vi "thermo_format_custom_values.vi"(0 "temp":dbl, 1 "format prefix":string, 2 "RH":dbl, 3 "press":dbl, 4 "channel":T1={"stat"=enum."Disabled", "type"=enum."COMET Tx5xx (ethernet)", "comment"="", "tag"="", "refresh"=5.0, "IP"="", "port"=502, "VISA"="", "last readout"=timestamp(0 s since 1904-01-01), "TCP ref"=refnum, "VISA sess"="", "idn"="", "press"=0.0, "RH"=0.0, "temp"=0.0, "pres cor"=[], "RH cor"=[], "temp cor"=[], "try left"=0, "failed"=FALSE, "RTD set"=[], "RTD inv"=[], "range"=0.0, "net mode"=enum."MODBUS"} {"RTD inv" format="%.1f"; "RTD set" format="%.1f"; "temp cor" format="%.1f"; "RH cor" format="%.1f"; "pres cor" format="%.1f"; "refresh" min=0.1 max=1000.0 format="%.2f"}, 5 "force print":bool) -> (6 "temperature":string, 7 "relh":string, 9 "pressure":string)   [LabVIEW 2013]
uses:
  thermo.ctl
  thermo_types.ctl
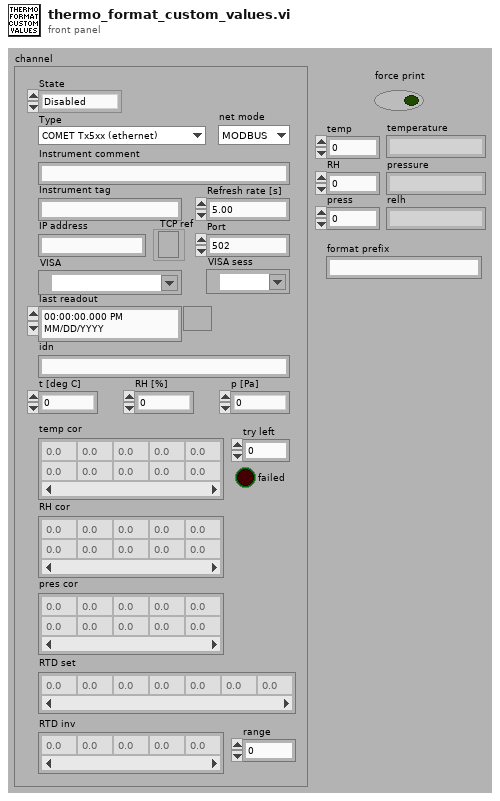
[diagram p1: front panel]
types:
  T1 = typedef "thermo.ctl" = cluster{"stat":enum16{"Disabled", "Enabled"}, "type":T2, "comment":string, "tag":string, "refresh":dbl, "IP":string, "port":u16, "VISA":refnum<visa-resource-name>, "last readout":timestamp, "TCP ref":refnum<k5>, "VISA sess":refnum<visa-resource-name>, "idn":string, "press":dbl, "RH":dbl, "temp":dbl, "pres cor":dbl[][], "RH cor":dbl[][], "temp cor":dbl[][], "try left":i32, "failed":bool, "RTD set":dbl[], "RTD inv":dbl[], "range":dbl, "net mode":enum16{"MODBUS", "HTTP"}}
  T2 = typedef "thermo_types.ctl" = enum16{"COMET Tx5xx (ethernet)", "Keithley 2002 (GPIB) + RTD", "Agilent 344xx (GPIB) + RTD"}
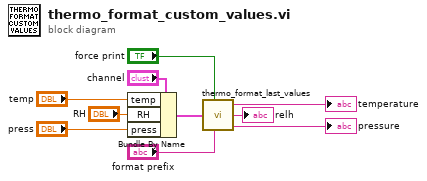
[diagram p0: block diagram]
diagram:
  n1 = Bundle By Name(cluster="channel", "temp"="temp", "RH"="RH", "press"="press") -> (w9:T1)
  n2 = call "thermo_format_last_values.vi"("force print"="force print", "thermo"=w9, "format prefix"="format prefix") -> ("temperature"=→"temperature":string, "RH"=→"relh":string, "pressure"=→"pressure":string)  [unwired: 2 in]
